vi "InApproachManeuverMode.vi"(11 "DistanceToNextWaypoint (m)":dbl) -> (3 "InApproachManeuverMode?":bool)   [LabVIEW 2013]
doc: "Theory: Within a certain distance from a waypoint, the boat should stop trying to do luff balancing and sail balancing, and should instead fall back on a simple relative wind to sail lookup (WindToSailLookup.vi). This should make the behavior around waypoints more predictable. The boat also shouldn't try using the sails to turn the boat for waypoint maneuvers, at least until we have tested the 'turn boat with sails' code wuite a bit.\n\nThis code simply reports 'Approaching Maneuver = TRUE' when the distance to the next waypoint dips below a cutoff value assigned as a default value in the VI.\n\nEric Schneider, Jan. 2014"
panel:
  in  "CutoffDistanceOfAlgorithm (m)":dbl=4.0
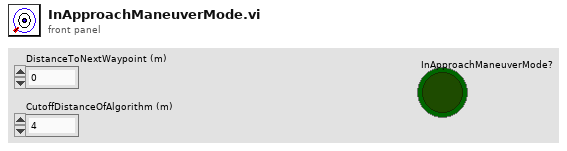
[diagram p1: front panel]
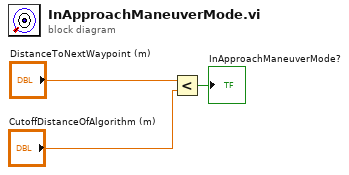
[diagram p0: block diagram]
diagram:
  n1 = Less?(x="DistanceToNextWaypoint (m)", y="CutoffDistanceOfAlgorithm (m)") -> (x < y?=→"InApproachManeuverMode?":bool)
